vi "test_TDMS File Integrity.vi"(8 "error in (no error)":errorcluster, 11 "TestCase in":refnum<class "Telemetry System Tests.lvclass">=refnum) -> (0 "error out":errorcluster, 3 "TestCase out":refnum<class "Telemetry System Tests.lvclass">)   [LabVIEW 2026, in "Telemetry System Tests.lvclass"]
uses:
  Telemetry System Tests.lvclass
  Telemetry System Tests.lvclass/Telemetry System Tests.ctl
  Telemetry Test Utilities/Telemetry Test Utilities.lvlib
  b15e678b-00b4-460c-84a3-511904b6b81c.vi
  3ba122ce-87e8-4d5d-9fcd-2cc66d275065.vi
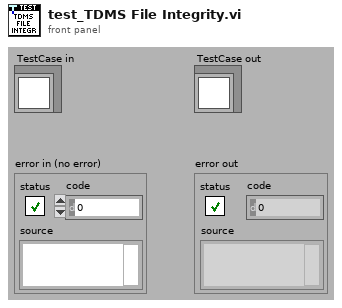
[diagram p1: front panel]
types:
  T1 = typedef "VeriStandTestUtilities.lvlib/TargetInformation.ctl" = cluster{"Name":string, "IP Address":string, "Operating System":string, "Target Rate":dbl, "Chassis List":T2[], "Custom Device List":string[]}
  T2 = typedef "VeriStandTestUtilities.lvlib/ChassisInformation.ctl" = cluster{"Name":string, "Devices":string[]}
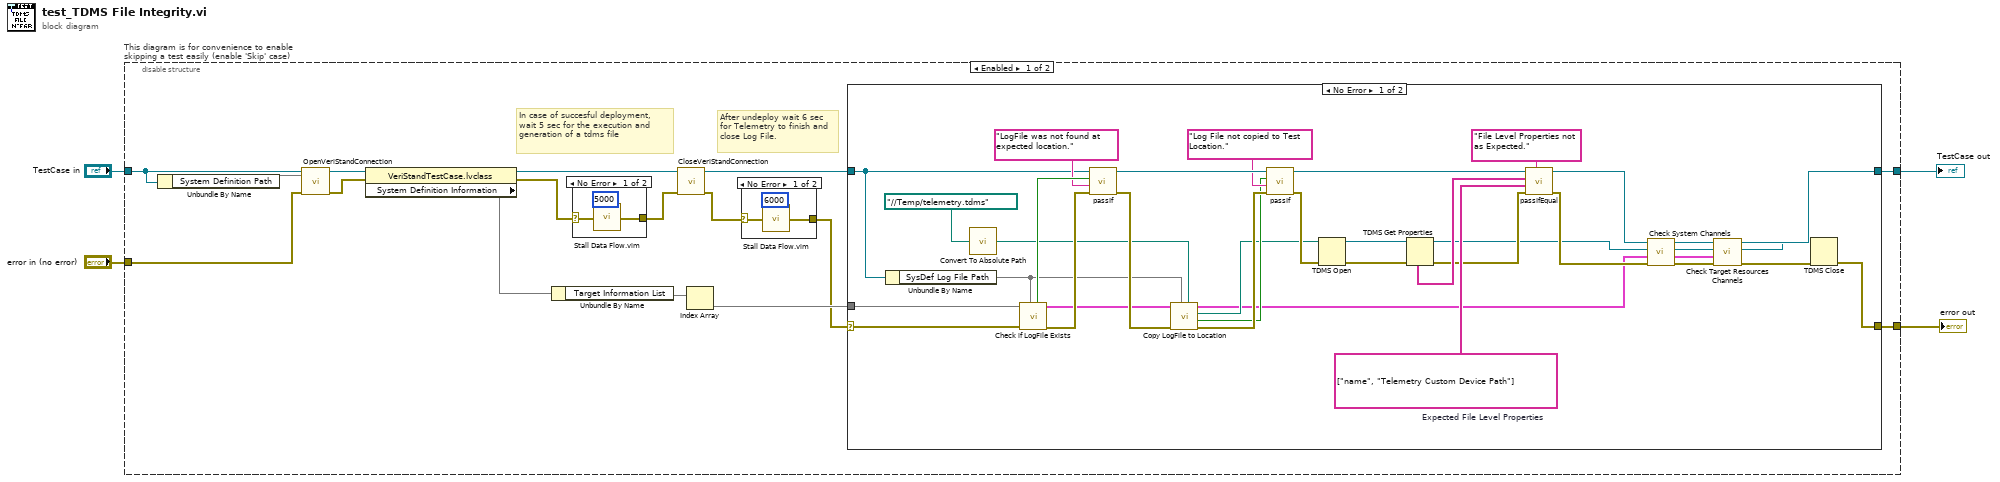
[diagram p0: block diagram]
diagram:
  n1 = disable-structure "This diagram is for convenience to enable skipping a test easily (enable 'Skip' case)" shown="Enabled" {
    disable-tunnel: "TestCase in" -> [w8 w70]
    disable-tunnel: [w19 w68] -> w1
    disable-tunnel: [w20 w69] -> w3
    disable-tunnel: "error in (no error)" -> [w18 w67]
    frame Enabled {
      # "After undeploy wait 6 sec for Telemetry to finish and close Log File."
      # "In case of succesful deployment, wait 5 sec for the execution and generation of a tdms file"
      n2 = Unbundle By Name(w8) -> ("System Definition Path"=w15)
      n3 = call-dynamic "OpenVeriStandConnection.vi"("error in (no error)"=w18, "System Definition File"=w15, "VeriStand Test Case in"=w8) -> ("error out"=w12:errorcluster, "VeriStand Test Case out"=w14:refnum<class "VeriStandTestCase.lvclass">)  [unwired: 6 in, 1 out]
      n4 = property class="VeriStandTestCase.lvclass"(reference=w14, error in=w12) -> (reference out=w13:refnum<class "VeriStandTestCase.lvclass">, error out=w7:errorcluster, "System Definition Information"=w11)
      n5 = Unbundle By Name(w11) -> ("Target Information List"=w10)
      n6 = case shown="No Error" w7 {
        selector: w7 -> [w27 w28]
        tunnel: [w25 w28] -> w16
        frame No Error {
          n7 = call "Stall Data Flow.vim"("value in"=w27, "milliseconds to wait"=u32 5000) -> ("value out"=w25:errorcluster)  [unwired: 1 out]
        }
        frame Error {
        }
      }
      n8 = call-dynamic "CloseVeriStandConnection.vi"("error in (no error)"=w16, "VeriStand Test Case in"=w13) -> ("error out"=w6:errorcluster, "VeriStand Test Case out"=w17:refnum<class "VeriStandTestCase.lvclass">)  [unwired: 8 in]
      n9 = Index Array(array=w10) -> (element=w9)  [unwired: 1 in]
      n10 = case shown="No Error" w6 {
        selector: w6 -> [w23 w24]
        tunnel: [w21 w24] -> w5
        frame No Error {
          n11 = call "Stall Data Flow.vim"("value in"=w23, "milliseconds to wait"=u32 6000) -> ("value out"=w21:errorcluster)  [unwired: 1 out]
        }
        frame Error {
        }
      }
      n12 = case shown="No Error" w5 {
        selector: w5 -> [w60 w66]
        tunnel: [w55 w66] -> w20
        tunnel: [w35 w65] -> w19
        tunnel: w17 -> [w49 w65]
        tunnel: w9 -> [w52 _]
        frame No Error {
          w46 = string[] ["name", "Telemetry Custom Device Path"]  # Expected File Level Properties
          n13 = Unbundle By Name(w49) -> ("SysDef Log File Path"=w50)
          n14 = call "Convert To Absolute Path.vi"("System Definition File Path"=path "../../Temp/telemetry.tdms" ("relative base path")) -> ("Absolute path"=w56:path)
          n15 = call "Check if LogFile Exists.vi"("Log File Path"=w50, "error in (no error)"=w60, "Target Information"=w52) -> ("error out"=w64:errorcluster, "Target Information out"=w51:T1, "LogFile Exists?"=w63:bool)  [unwired: 6 in]
          n16 = call-dynamic "passIf.vi"("error in (no error)"=w64, "message (\"\")"="LogFile was not found at expected location." ("message (\"\")"), "pass"=w63, "TestCase in"=w49) -> ("error out"=w62:errorcluster, "TestCase out"=w59:refnum<class "Telemetry System Tests.lvclass">)  [unwired: 6 in]
          n17 = call "Copy LogFile to Location.vi"("Local Save Path in"=w56, "Log File Path in"=w50, "error in"=w62, "Target Information in"=w51) -> ("error out"=w58:errorcluster, "File Succesfuly copied"=w32:bool, "Local Save Path out"=w31:path, "Target Information out"=w30:T1)  [unwired: 4 in]
          n18 = call-dynamic "passIf.vi"("error in (no error)"=w58, "message (\"\")"="Log File not copied to Test Location." ("message (\"\")"), "pass"=w32, "TestCase in"=w59) -> ("error out"=w57:errorcluster, "TestCase out"=w44:refnum<class "Telemetry System Tests.lvclass">)  [unwired: 6 in]
          n19 = TDMS Open(8:w57, 11:w31) -> (0:w42:errorcluster, 3:w43:refnum<k34>)  [unwired: 5 in]
          n20 = TDMS Get Properties(8:w42, 11:w43) -> (0:w45:errorcluster, 3:w40:refnum<k34>, 6:w48:string[])  [unwired: 4 in, 3 out]
          n21 = call-dynamic "passIfEqual.vi"("custom report message (\"\")"="File Level Properties not as Expected." ("custom report message (\"\")"), "error in (no error)"=w45, "y"=w46, "x"=w48, "TestCase in"=w44) -> ("error out"=w41:errorcluster, "TestCase out"=w39:refnum<class "Telemetry System Tests.lvclass">)  [unwired: 5 in]
          n22 = call "Check System Channels.vi"("error in"=w41, "Target Information in"=w30, "tdms file in"=w40, "Telemetry System Tests in"=w39) -> ("error out"=w37:errorcluster, "Target Information out"=w29:T1, "tdms file out"=w36:refnum<k34>, "Telemetry System Tests out"=w38:refnum<class "Telemetry System Tests.lvclass">)  [unwired: 4 in]
          n23 = call "Check Target Resources Channels.vi"("error in"=w37, "Target Information in"=w29, "tdms file in"=w36, "Telemetry System Tests in"=w38) -> ("error out"=w33:errorcluster, "tdms file out"=w34:refnum<k34>, "Telemetry System Tests out"=w35:refnum<class "Telemetry System Tests.lvclass">)  [unwired: 4 in, 1 out]
          n24 = TDMS Close(8:w33, 11:w34) -> (0:w55:errorcluster)  [unwired: 1 out]
        }
        frame Error {
        }
      }
    }
    frame Disabled {
      # "skip test result while test is under development"
      n25 = call <vilib>:"skip.vi"("error in (no error)"=w67, "TestCase in"=w70) -> ("error out"=w69:errorcluster, "TestCase out"=w68:refnum<class "Telemetry System Tests.lvclass">)  [unwired: 8 in]
    }
  }
  "error out" <- w3
  "TestCase out" <- w1
